vi "Motor_Init.vi"(8 "error in":errorcluster, 11 "FPGA_Ref_in":refnum<k20>) -> (0 "error out":errorcluster, 3 "FPGA_Ref_out":refnum<k20>)   [LabVIEW 2009, in "Motor.lvlib"]
uses:
  Motor.lvlib
  PWM/PWM_Name.ctl
  PWM.lvlib
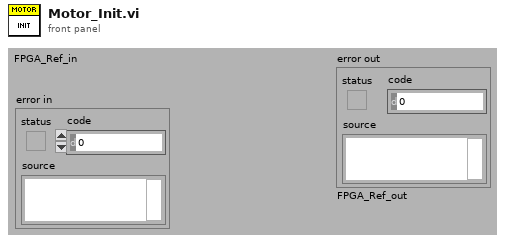
[diagram p1: front panel]
types:
  T1 = typedef "PWM.lvlib/PWM_Name.ctl" = u16
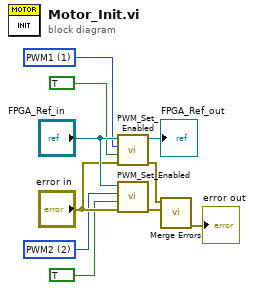
[diagram p0: block diagram]
diagram:
  w3 = T1 2 items=["Invalid"=0, "PWM1"=1, "PWM2"=2, "PWM9"=9, "PWM10"=10] ("PWM_in")
  w4 = T1 1 items=["Invalid"=0, "PWM1"=1, "PWM2"=2, "PWM9"=9, "PWM10"=10] ("PWM_in")
  n1 = call "PWM_Set_Enabled.vi"("error in"="error in", "Enable"=TRUE, "PWM_in"=w4, "FPGA_Ref_in"="FPGA_Ref_in") -> ("error out"=w9:errorcluster, "FPGA_Ref_out"=→"FPGA_Ref_out":refnum<k20>)  [unwired: 5 in, 1 out]
  n2 = call "PWM_Set_Enabled.vi"("error in"="error in", "Enable"=TRUE, "PWM_in"=w3, "FPGA_Ref_in"="FPGA_Ref_in") -> ("error out"=w8:errorcluster)  [unwired: 5 in, 2 out]
  n3 = call <vilib>:"Merge Errors.vi"("error in 2 (no error)"=w8, "error in 1 (no error)"=w9) -> ("error out"=→"error out":errorcluster)  [unwired: 5 in]
